vi "Create DAQmx Task.vi"(8 "error in (no error)":errorcluster, 11 "DAQmxDI in":refnum<class "DAQmxDI.lvclass">) -> (0 "error out":errorcluster, 3 "DAQmxDI out":refnum<class "DAQmxDI.lvclass">)   [LabVIEW 2023, in "VolatusDAQ.lvlib" / "DAQmxDI.lvclass"]
uses:
  DAQmxDI.lvclass
  DAQmxDI.lvclass/DAQmxDI.ctl
  Volatus/Module/Module.lvclass
  VolatusConfig/Task/Task Config.lvclass
  VolatusConfig/VolatusConfigElement/VolatusConfigElement.lvclass
  VolatusDAQConfig/VolatusDAQConfig.lvlib
  lv-vecto/Vecto/Group DBL/Group DBL.lvclass
  VolatusDAQ.lvlib
  <resource>/objmgr/daqmx.rc
  <vilib>/DAQmx/create/channels.llb/DAQmx Create Channel (DI-Digital Input).vi
  lv-cdm/CDM-Config/Config Element/Config Element.lvclass
  <vilib>/DAQmx/configure/timing.llb/DAQmx Timing (Sample Clock).vi
  VolatusConfig/Group/Group Config.lvclass
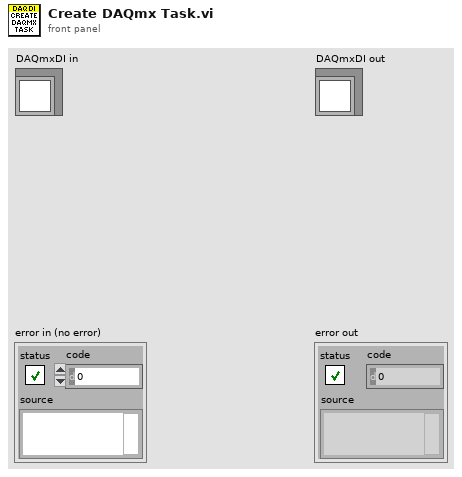
[diagram p1: front panel]
types:
  T1 = typedef "VolatusDAQ.lvlib/DAQmxDI.lvclass/Port Info.ctl" = cluster{"Module Alias":string, "Number":i32, "# Lines":i32, "Lines":map{i32, string}, "Channel Indices":i32[]}
  T2 = typedef "VolatusDAQConfig.lvlib/Sampling Config.ctl" = cluster{"Rate":dbl, "Chunk Size":i32}
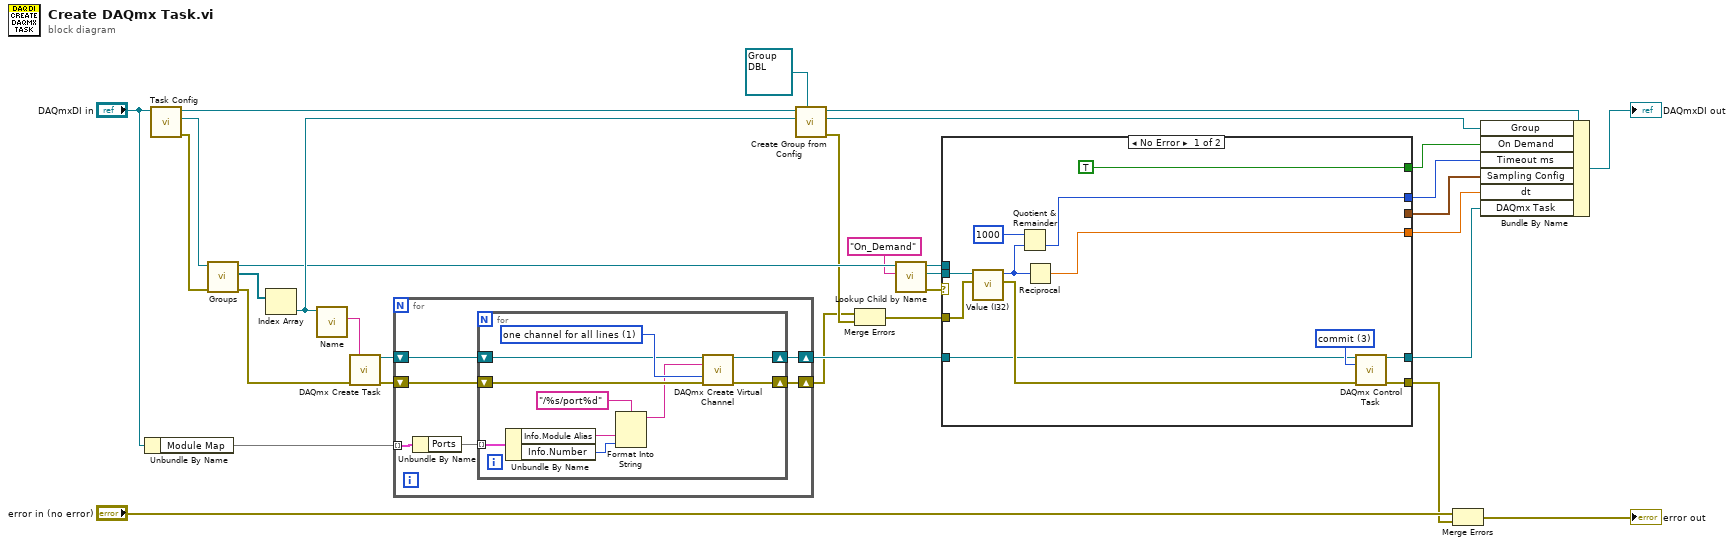
[diagram p0: block diagram]
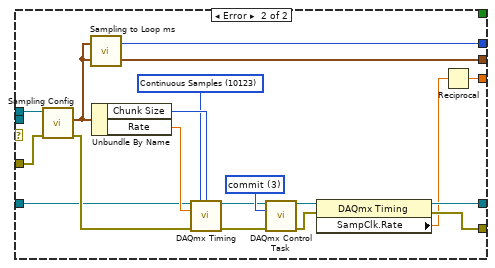
[diagram p2: hidden frame]
diagram:
  n1 = Unbundle By Name("DAQmxDI in") -> ("Module Map"=w22:map{string, map{i32, T1}})
  n2 = call "Task Config.vi"("Module in"="DAQmxDI in") -> ("error out"=w30:errorcluster, "Task Config"=w29:refnum<class "Task Config.lvclass">, "Module out"=w26:refnum<class "DAQmxDI.lvclass">)  [unwired: 8 in]
  n3 = call "Groups.vi"("error in (no error)"=w30, "Task in"=w29) -> ("error out"=w32:errorcluster, "Groups"=w28:refnum<class "Group Config.lvclass">[], "Task out"=w11:refnum<class "Task Config.lvclass">)  [unwired: 7 in]
  n4 = Index Array(array=w28) -> (element=w17:refnum<class "Group Config.lvclass">)  [unwired: 1 in]
  n5 = call "Name.vi"("VolatusConfigElement in"=w17) -> ("Name"=w25:string)  [unwired: 8 in, 2 out]
  n6 = call <vilib>:"DAQmx Create Task.vi"("new task name"=w25, "error in"=w32) -> ("task out"=w24:refnum<k21>, "error out"=w23:errorcluster)  [unwired: 12 in]
  n7 = for {
    shift-right: [w34] -> w21
    shift-left: w24 -> [w35]
    shift-right: [w33] -> w7
    shift-left: w23 -> [w36]
    tunnel: w22 -> [w38] mode=indexing
    n8 = Unbundle By Name(w38) -> ("Ports"=w37:map{i32, T1})
    n9 = for {
      tunnel: w37 -> [w48] mode=indexing
      shift-right: [w40] -> w33
      shift-left: w36 -> [w42]
      shift-right: [w39] -> w34
      shift-left: w35 -> [w43]
      w44 = 1 items=["one channel for each line", "one channel for all lines"] ("line grouping")
      n10 = Unbundle By Name(w48) -> ("Info.Module Alias"=w46:string, "Info.Number"=w45:i32)
      n11 = Format Into String(format string="/%s/port%d", w46, w45) -> (resulting string=w41:string)  [unwired: 2 in, 1 out]
      n12 = call-poly <vilib>:"DAQmx Create Virtual Channel.vi"("task in"=w43, "lines"=w41, "line grouping"=w44, "error in"=w42) -> ("task out"=w39:refnum<k21>, "error out"=w40:errorcluster)  [unwired: 10 in]
    }
  }
  n13 = call "Create Group from Config.vi"("Group Type (Abstract)"=refnum<class "Group DBL.lvclass"> refnum ("Vecto.lvlib:Group DBL.lvclass"), "Group Config"=w17, "Module in"=w26) -> ("error out"=w8:errorcluster, "Group"=w15:refnum<class "Group DBL.lvclass">, "Module out"=w18:refnum<class "DAQmxDI.lvclass">)  [unwired: 6 in]
  n14 = Merge Errors(w7, w8) -> (w6:errorcluster)
  n15 = call "Lookup Child by Name.vi"("Child Name"="On_Demand", "VolatusConfigElement in"=w11) -> ("error out"=w12:errorcluster, "Child"=w5:refnum<class "Config Element.lvclass">, "VolatusConfigElement out"=w10:refnum<class "Task Config.lvclass">)  [unwired: 6 in, 1 out]
  n16 = case shown="No Error" w12 {
    tunnel: w21 -> [w53 w73]
    tunnel: [w55 w65] -> w3
    tunnel: [w54 w78] -> w2
    tunnel: [w51 w72] -> w14
    tunnel: [_ w71] -> w13
    tunnel: w10 -> [_ w70]
    tunnel: w6 -> [w58 w69]
    tunnel: w5 -> [w59 _]
    tunnel: [TRUE _] -> w4
    tunnel: [w49 w64] -> w1
    frame No Error {
      w56 = 3 items=["verify"=2, "reserve"=4, "commit"=3, "unreserve"=5, "abort"=6] ("action")
      n17 = call "Value (I32).vi"("error in (no error)"=w58, "Config Element in"=w59) -> ("error out"=w60:errorcluster, "I32 Value"=w50:i32)  [unwired: 8 in]
      n18 = Quotient & Remainder(x=1000 ("y"), y=w50) -> (floor(x/y)=w51:i32)  [unwired: 1 out]
      n19 = Reciprocal(x=w50) -> (1/x=w49:dbl)
      n20 = call <vilib>:"DAQmx Control Task.vi"("task/channels in"=w53, "action"=w56, "error in"=w60) -> ("task out"=w55:refnum<k21>, "error out"=w54:errorcluster)  [unwired: 11 in]
    }
    frame Error {
      w66 = 3 items=["verify"=2, "reserve"=4, "commit"=3, "unreserve"=5, "abort"=6] ("action")
      w74 = 10123 items=["Finite Samples"=10178, "Continuous Samples"=10123, "Hardware Timed Single Point"=12522] ("sample mode")
      n21 = call "Sampling Config.vi"("error in (no error)"=w69, "Task In"=w70) -> ("error out"=w77:errorcluster, "Sampling Config"=w71:T2)  [unwired: 7 in, 1 out]
      n22 = call "Sampling to Loop ms.vi"("Sampling Config"=w71) -> ("Loop Timeout ms"=w72:i32)  [unwired: 6 in]
      n23 = Unbundle By Name(w71) -> ("Chunk Size"=w75:i32, "Rate"=w76:dbl)
      n24 = call-poly <vilib>:"DAQmx Timing.vi"("task/channels in"=w73, "sample mode"=w74, "samples per channel"=w75, "rate"=w76, "error in"=w77) -> ("task out"=w62:refnum<k21>, "error out"=w61:errorcluster)  [unwired: 9 in]
      n25 = call <vilib>:"DAQmx Control Task.vi"("task/channels in"=w62, "action"=w66, "error in"=w61) -> ("task out"=w67:refnum<k21>, "error out"=w68:errorcluster)  [unwired: 11 in]
      n26 = property class="DAQmx Timing"(reference=w67, error in=w68) -> (reference out=w65:refnum<k21>, error out=w78:errorcluster, "SampClk.Rate"=w63:dbl)
      n27 = Reciprocal(x=w63) -> (1/x=w64:dbl)
    }
  }
  n28 = Merge Errors("error in (no error)", w2) -> (→"error out":errorcluster)
  n29 = Bundle By Name(cluster=w18, "Group"=w15, "On Demand"=w4, "Timeout ms"=w14, "Sampling Config"=w13, "dt"=w1, "DAQmx Task"=w3) -> (→"DAQmxDI out":refnum<class "DAQmxDI.lvclass">)
